vi "Sift Proxy Smoketest.vi"() -> ()   [LabVIEW 2024]
doc: "Smoketest for Sift Proxy. This example verifies that Sift Proxy is installed correctly."
uses:
  Sift API/Sift Client.lvclass
panel:
  in  "Log Path":path
  out "VI Progress":i32(slide) scale=0.0..1000.0
  out "Error":errorcluster
  in  "Organization ID":string
  in  "API Key":string
  in  "API URL":string
  # "Sift Proxy Smoketest"
  # "Instructions\n\n1. Fill in the API URL, API Key, and Organization ID. Visit this URL for more information on authentication\n    https://docs.siftstack.com/docs/api/authentication\n\n    Fill in a  Log path. The Log path is there Sift Proxy logs will be stored.\n\n2. Start the VI\n\n3. Navigate to the Assets page and look for an asset titled \"sift-proxy-X\" where X is your host name.\n\n4. You should see the Sift Proxy asset and metrics telemetry in this view.\n\n5. Wait for a few seconds and the VI should automatically exit."
  # "This example verifies that Sift Proxy is installed correctly for streaming."
  # "The application will stream metrics for 10s before stopping."
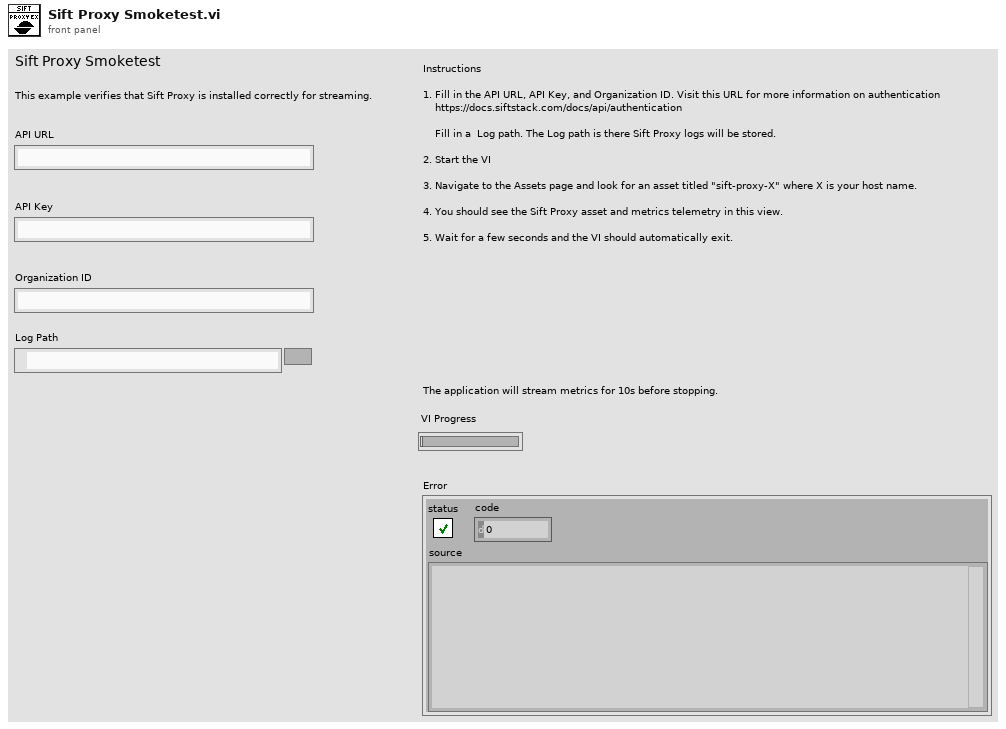
[diagram p1: front panel]
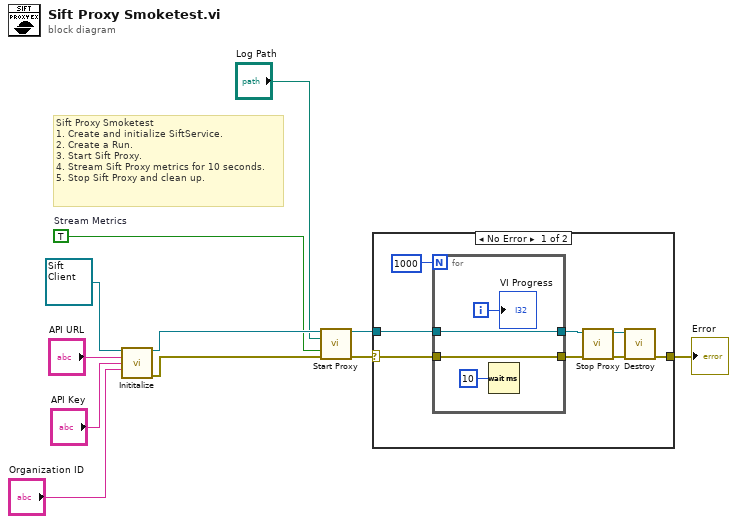
[diagram p0: block diagram]
diagram:
  w5 = TRUE  # Stream Metrics
  # "Sift Proxy Smoketest\n1. Create and initialize SiftService.\n2. Create a Run.\n3. Start Sift Proxy.\n4. Stream Sift Proxy metrics for 10 seconds.\n5. Stop Sift Proxy and clean up."
  n1 = call-dynamic "Inititalize.vi"("Sift Client in"=refnum<class "Sift Client.lvclass"> refnum ("Sift Client.lvlib:Sift Client.lvclass"), "API URL"="API URL", "API Key"="API Key", "Organization ID"="Organization ID") -> ("Sift Client out"=w7:refnum<class "Sift Client.lvclass">, "error out"=w6:errorcluster)  [unwired: 10 in]
  n2 = call-dynamic "Start Proxy.vi"("Sift Client in"=w7, "Storage Path"="Log Path", "Stream Metrics"=w5, "error in (no error)"=w6) -> ("Sift Client out"=w4:refnum<class "Sift Client.lvclass">, "error out"=w3:errorcluster)  [unwired: 10 in]
  n3 = case shown="No Error" w3 {
    selector: w3 -> [w13 w24]
    tunnel: w4 -> [w17 _]
    tunnel: [w12 w24] -> w2
    frame No Error {
      n4 = for {
        N: 1000 -> [_]
        tunnel: [w22] -> w18
        tunnel: w17 -> [w22]
        tunnel: [w21] -> w16
        tunnel: w13 -> [w21]
        i -> [w20]
        n5 = Wait (ms)(milliseconds to wait=u32 10) -> ()  [unwired: 1 out]
        "VI Progress" <- w20
      }
      n6 = call-dynamic "Stop Proxy.vi"("error in (no error)"=w16, "Sift Client in"=w18) -> ("error out"=w15:errorcluster, "Sift Client out"=w14:refnum<class "Sift Client.lvclass">)  [unwired: 7 in, 1 out]
      n7 = call-dynamic "Destroy.vi"("error in (no error)"=w15, "Sift Client in"=w14) -> ("error out"=w12:errorcluster)  [unwired: 8 in, 1 out]
    }
    frame Error {
    }
  }
  "Error" <- w2
